vi "LabvolutionSubmoduleCheck_GitSubmoduleAdd.vi"(8 "error in (no error)":errorcluster, 10 "Repository URL":string, 11 "Folder in":path) -> (0 "error out":errorcluster, 2 "Command OK":bool, 3 "Working Dir out":path)   [LabVIEW 2018]
uses:
  callback-system-exec/callback-system-exec/callback-system-exec.lvlib
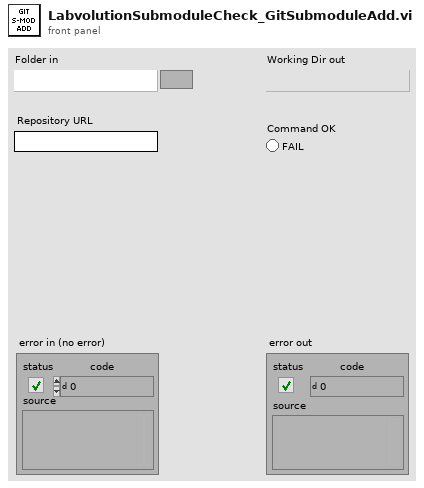
[diagram p1: front panel]
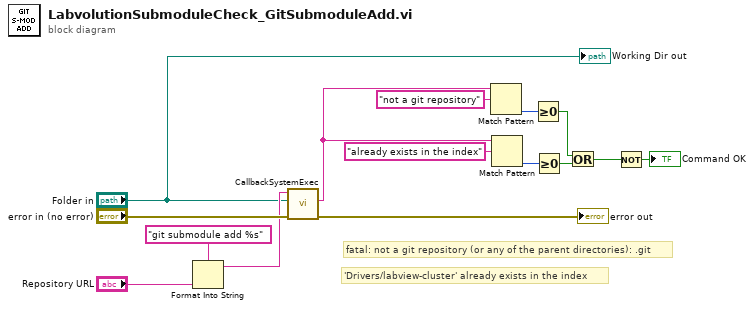
[diagram p0: block diagram]
diagram:
  # "'Drivers/labview-cluster' already exists in the index"
  # "fatal: not a git repository (or any of the parent directories): .git"
  n1 = Format Into String(format string="git submodule add %s", "Repository URL") -> (resulting string=w2:string)  [unwired: 2 in, 1 out]
  n2 = call "CallbackSystemExec.vi"("error in (no error)"="error in (no error)", "Working directory"="Folder in", "Command"=w2) -> ("error out"=→"error out":errorcluster, "Standard Error"=w3:string)  [unwired: 6 in, 1 out]
  n3 = Match Pattern(string=w3, regular expression="not a git repository") -> (offset past match=w14:i32)  [unwired: 1 in, 3 out]
  n4 = Match Pattern(string=w3, regular expression="already exists in the index") -> (offset past match=w8:i32)  [unwired: 1 in, 3 out]
  n5 = Greater Or Equal To 0?(x=w14) -> (x >= 0?=w10:bool)
  n6 = Greater Or Equal To 0?(x=w8) -> (x >= 0?=w6:bool)
  n7 = Or(x=w10, y=w6) -> (x .or. y?=w9:bool)
  n8 = Not(x=w9) -> (.not. x?=→"Command OK":bool)
  "Working Dir out" <- "Folder in"
